vi "ServerOption.vi"(8 "error in":errorcluster, 9 "BD_Arch":refnum<vi>, 10 "BD_Op":refnum<vi>, 11 "Ring in":refnum<vi>) -> (0 "error out":errorcluster)   [LabVIEW 2019]
uses:
  Communication/TypeDef/#TypeDef_SetGet.ctl
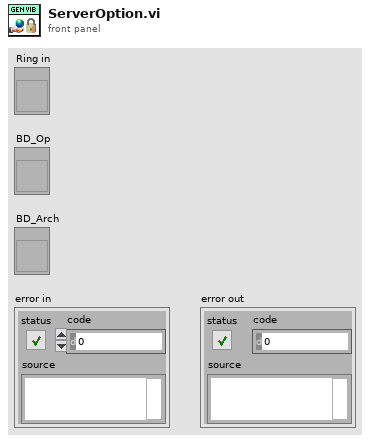
[diagram p1: front panel]
types:
  T1 = typedef "#TypeDef_SetGet.ctl" = enum16{"Set", "Get"}
  T2 = typedef "#TypeDef_DBMode.ctl" = u16
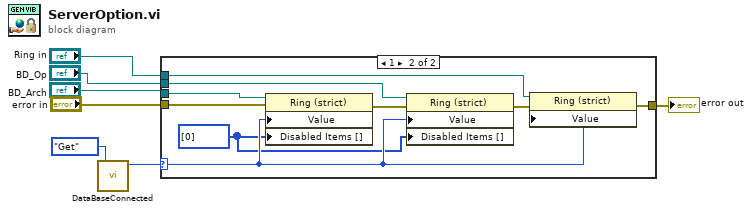
[diagram p0: block diagram]
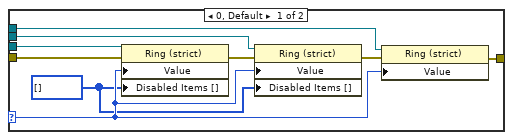
[diagram p2: hidden frame]
diagram:
  n1 = call "DataBaseConnected.vi"("Get/Set"=#TypeDef_SetGet."Get") -> ("BD out"=w4:T2)  [unwired: 10 in]
  n2 = case shown="1" w4 {
    selector: w4 -> [w13 w18]
    tunnel: "BD_Arch" -> [w16 w25]
    tunnel: "BD_Op" -> [w8 w23]
    tunnel: "Ring in" -> [w14 w20]
    tunnel: [w11 w19] -> w7
    tunnel: "error in" -> [w10 w22]
    frame 0, Default {
      w9 = i32[] [] ("Disabled Items []")
      n3 = property class="Ring (strict)"(reference=w16, error in=w10, "Value"=w13, "Disabled Items []"=w9) -> (error out=w12:errorcluster)  [unwired: 1 out]
      n4 = property class="Ring (strict)"(reference=w8, error in=w12, "Value"=w13, "Disabled Items []"=w9) -> (error out=w15:errorcluster)  [unwired: 1 out]
      n5 = property class="Ring (strict)"(reference=w14, error in=w15, "Value"=w13) -> (error out=w11:errorcluster)  [unwired: 1 out]
    }
    frame 1 {
      w17 = i32[] [0] ("Disabled Items []")
      n6 = property class="Ring (strict)"(reference=w25, error in=w22, "Value"=w18, "Disabled Items []"=w17) -> (error out=w24:errorcluster)  [unwired: 1 out]
      n7 = property class="Ring (strict)"(reference=w23, error in=w24, "Value"=w18, "Disabled Items []"=w17) -> (error out=w21:errorcluster)  [unwired: 1 out]
      n8 = property class="Ring (strict)"(reference=w20, error in=w21, "Value"=w18) -> (error out=w19:errorcluster)  [unwired: 1 out]
    }
  }
  "error out" <- w7
